vi "Write Get Meta Data.vi"(8 "error in":errorcluster, 10 "Get Meta Data":T1, 11 "UDP in":refnum<class "UDP.lvclass">) -> (0 "error out":errorcluster, 3 "UDP out":refnum<class "UDP.lvclass">)   [LabVIEW 2020, in "Plugin Instrument Driver.lvlib" / "UDP.lvclass"]
doc: "Get Meta Data"
uses:
  UDP.lvclass
  builds/Libraries/Shared GUI Library.lvlibp/Shared GUI Library/Device Meta Data Cluster/Get Meta Data.ctl
  UDP.lvclass/UDP.ctl
  builds/Libraries/Shared GUI Library.lvlibp
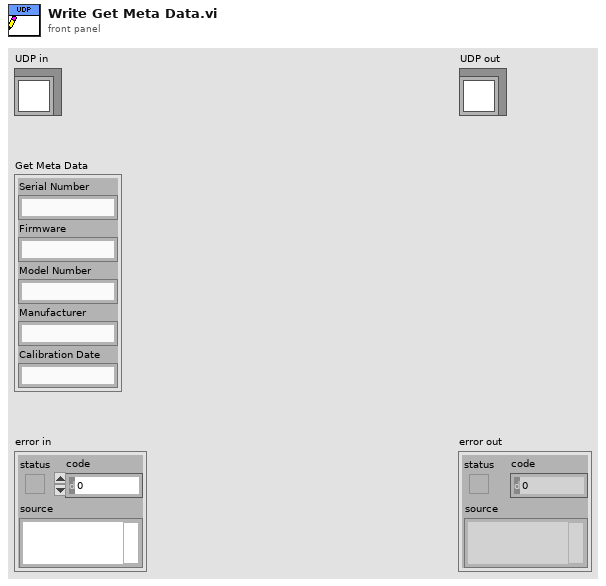
[diagram p1: front panel]
types:
  T1 = typedef "Shared GUI Library.lvlibp/Get Meta Data.ctl" = cluster{"Serial Number":string, "Firmware":string, "Model Number":string, "Manufacturer":string, "Calibration Date":string}
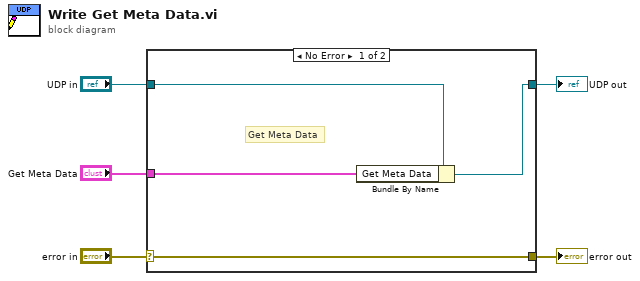
[diagram p0: block diagram]
diagram:
  n1 = case shown="No Error" "error in" {
    selector: "error in" -> [w9 w10]
    tunnel: [w9 w10] -> w4
    tunnel: [w7 w11] -> w2
    tunnel: "UDP in" -> [w8 w11]
    tunnel: "Get Meta Data" -> [w6 _]
    frame No Error {
      # "Get Meta Data"
      n2 = Bundle By Name(cluster=w8, "Get Meta Data"=w6) -> (w7:refnum<class "UDP.lvclass">)
    }
    frame Error {
    }
  }
  "error out" <- w4
  "UDP out" <- w2
